vi "Test write FITS 3D RGB.vi"() -> ()   [LabVIEW 2023]
uses:
  gfitsio.lvlib
  cfitsio-bitpix.ctl
  gfitsio-write-image-subset-variant.vi
panel:
  out "new picture":picture
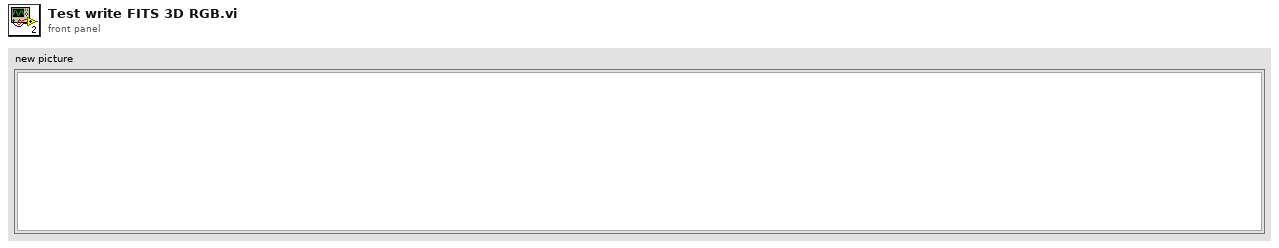
[diagram p1: front panel]
types:
  T1 = typedef "gfitsio.lvlib/cfitsio-bitpix.ctl" = i32
  T2 = typedef "gfitsio.lvlib/gfitsio-refnum.ctl" = refnum<k1>
  T3 = typedef "imagedata.ctl" = cluster{"image type":i32, "image depth":i32, "image":u8[], "mask":u8[], "colors":u32[], "Rectangle":cluster{"left":i16, "top":i16, "right":i16, "bottom":i16}}
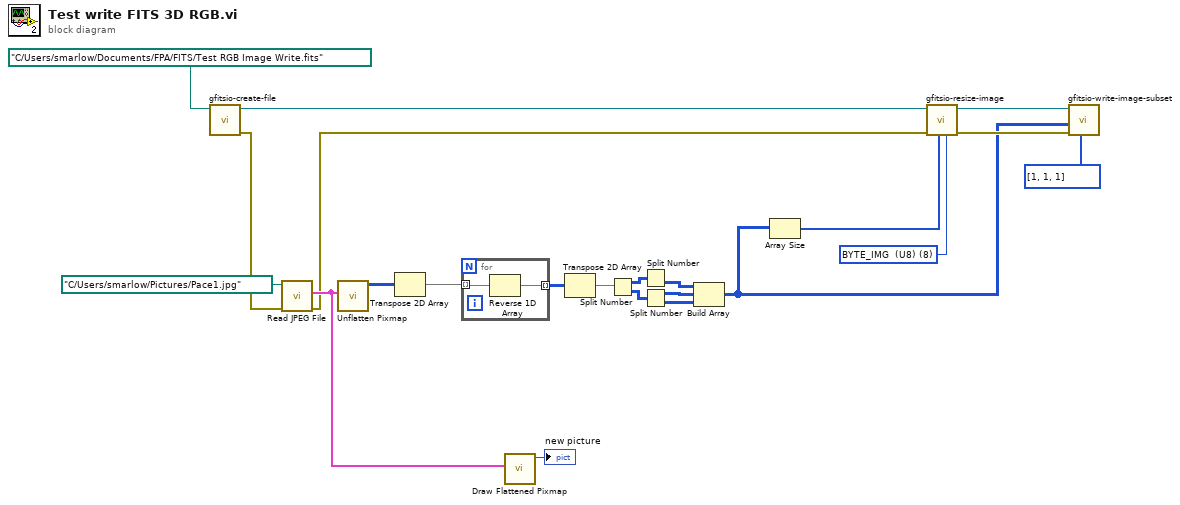
[diagram p0: block diagram]
diagram:
  w17 = T1 8 items=["<invalid type>"=0, "BYTE_IMG  (U8)"=8, "SHORT_IMG  (I16)"=16, "USHORT_IMG  (U16)"=20, "LONG_IMG  (I32)"=32, "ULONG_IMG  (U32)"=40, "FLOAT_IMG  (SGL)"=-32, "DOUBLE_IMG  (DBL)"=-64] ("image data type")
  n1 = call "gfitsio-create-file.vi"("path"=path "C:/Users/smarlow/Documents/FPA/FITS/Test RGB Image Write.fits") -> ("error out"=w19:errorcluster, "gfits refnum"=w21:T2)  [unwired: 9 in]
  n2 = call <vilib>:"Read JPEG File.vi"("error in (no error)"=w19, "path to JPEG file"=path "C:/Users/smarlow/Pictures/Pace1.jpg" ("path to PNG file")) -> ("error out"=w13:errorcluster, "image data"=w16:T3)  [unwired: 7 in, 1 out]
  n3 = call <vilib>:"Unflatten Pixmap.vi"("image data"=w16) -> ("24-bit pixmap"=w4:u32[][])  [unwired: 4 in, 6 out]
  n4 = Transpose 2D Array(2D array=w4) -> (transposed array=w3:u32[][])
  n5 = for {
    tunnel: w3 -> [w24] mode=indexing
    tunnel: [w23] -> w14 mode=indexing
    n6 = Reverse 1D Array(array=w24) -> (reversed array=w23:u32[])
  }
  n7 = call <vilib>:"Draw Flattened Pixmap.vi"("image data"=w16) -> ("new picture"=→"new picture":picture)  [unwired: 8 in]
  n8 = Transpose 2D Array(2D array=w14) -> (transposed array=w6:u32[][])
  n9 = Split Number(x=w6) -> (hi(x)=w7:u16[][], lo(x)=w8:u16[][])
  n10 = Split Number(x=w7) -> (lo(x)=w9:u8[][])  [unwired: 1 out]
  n11 = Split Number(x=w8) -> (hi(x)=w10:u8[][], lo(x)=w11:u8[][])
  n12 = Build Array(w9, w10, w11) -> (w2:u8[][][])
  n13 = Array Size(array=w2) -> (size(s)=w1:i32[])
  n14 = call "gfitsio-resize-image.vi"("image data type"=w17, "naxes"=w1, "error in (no error)"=w13, "gfits refnum"=w21) -> ("error out"=w18:errorcluster, "dup gfits refnum"=w12:T2)  [unwired: 6 in]
  n15 = call-poly "gfitsio-write-image-subset.vi"("fpixel"=i32[] [1, 1, 1], "error in (no error)"=w18, "data"=w2, "gfits refnum"=w12) -> ()  [unwired: 6 in, 2 out]
